vi "input.vi"(8 "error in":errorcluster, 10 "data table in":T1, 11 "TEC runtime in":refnum<class "TEC runtime.lvclass">) -> (0 "error out":errorcluster, 2 "data table out":T1, 3 "TEC runtime out":refnum<class "TEC runtime.lvclass">)   [LabVIEW 2013, in "TEC runtime.lvclass"]
doc: "Provides an interface for reading data from a module at runtime. While this interface performs no operations, a child should provide an override which may read from any open sessions, references, or interfaces."
uses:
  TEC runtime.lvclass
  <vilib>/NI/Tag Bus/table/data table.ctl
  TEC runtime.lvclass/TEC runtime.ctl
  <vilib>/NI/Tag Bus/table/data table.lvlib
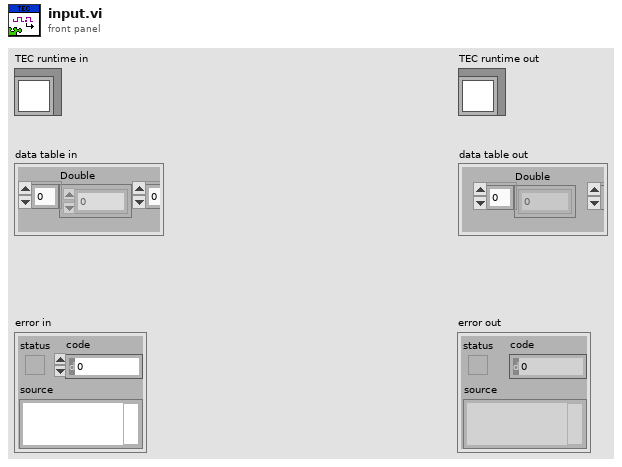
[diagram p1: front panel]
types:
  T1 = typedef "tag bus.lvlib/data table.lvlib/data table.ctl" = cluster{"Double":dbl[], "Single":sgl[], "I64":i64[], "I32":i32[], "I16":i16[], "I8":i8[], "U64":u64[], "U32":u32[], "U16":u16[], "U8":u8[], "Boolean":bool[], "String":string[], "Array of Double":cluster{"DBL Array":dbl[]}[], "Array of Single":cluster{"SGL Array":sgl[]}[], "Array of I64":cluster{"I64 Array":i64[]}[], "Array of I32":cluster{"I32 Array":i32[]}[], "Array of I16":cluster{"I16 Array":i16[]}[], "Array of I8":cluster{"I8 Array":i8[]}[], "Array of U64":cluster{"U64 Array":u64[]}[], "Array of U32":cluster{"U32 Array":u32[]}[], "Array of U16":cluster{"U16 Array":u16[]}[], "Array of U8":cluster{"U8 Array":u8[]}[], "Array of Boolean":cluster{"Boolean Array":bool[]}[], "Array of String":cluster{"String Array":string[]}[]}
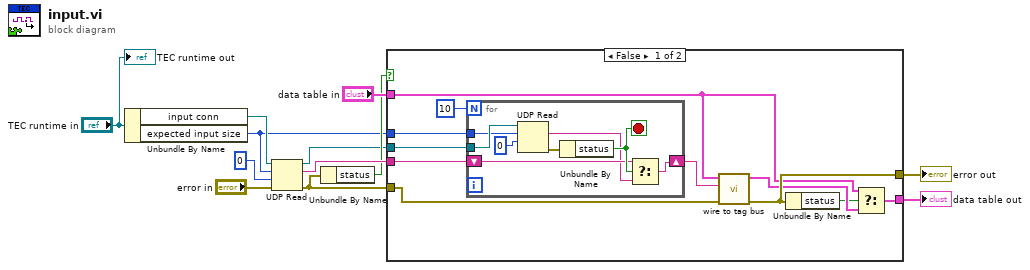
[diagram p0: block diagram]
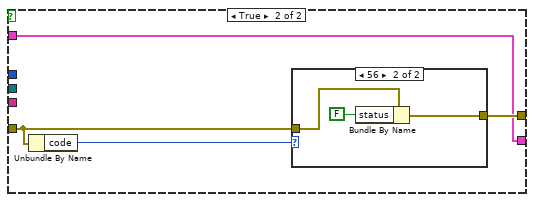
[diagram p2: hidden frame]
diagram:
  n1 = Unbundle By Name("TEC runtime in") -> ("input conn"=w11:refnum<k16>, "expected input size"=w1:i32)
  n2 = UDP Read(connection ID=w11, max size (548)=w1, timeout ms (25000)=0, 8:"error in") -> (data out=w5:string, error out=w3:errorcluster, 3:w2:refnum<k16>)  [unwired: 2 out]
  n3 = Unbundle By Name(w3) -> ("status"=w4:bool)
  n4 = case shown="False" w4 {
    tunnel: "data table in" -> [w20 w32]
    tunnel: [w23 w33] -> w7
    tunnel: [w21 w32] -> w6
    tunnel: w5 -> [w18 _]
    tunnel: w3 -> [w13 w34]
    tunnel: w2 -> [w15 _]
    tunnel: w1 -> [w14 _]
    frame False {
      n5 = for {
        N: 10 -> [_]
        shift-right: [w25] -> w17
        shift-left: w18 -> [w26]
        tunnel: w15 -> [w31]
        tunnel: w14 -> [w30]
        stop <- w27 stop-if-true
        n6 = UDP Read(connection ID=w31, max size (548)=w30, timeout ms (25000)=0) -> (data out=w24:string, error out=w28:errorcluster)  [unwired: 1 in, 3 out]
        n7 = Unbundle By Name(w28) -> ("status"=w27:bool)
        n8 = Select(t=w26, s=w27, f=w24) -> (s? t:f=w25:string)
      }
      n9 = call "wire to tag bus.vi"("error in"=w13, "wire data"=w17, "data table in"=w20) -> ("error out"=w23:errorcluster, "data table out"=w22:T1)  [unwired: 7 in]
      n10 = Unbundle By Name(w23) -> ("status"=w16:bool)
      n11 = Select(t=w20, s=w16, f=w22) -> (s? t:f=w21:T1)
    }
    frame True {
      n12 = Unbundle By Name(w34) -> ("code"=w35:i32)
      n13 = case shown="56" w35 {
        tunnel: w34 -> [w36 w39]
        tunnel: [w36 w37] -> w33
        frame Default {
        }
        frame 56 {
          n14 = Bundle By Name(cluster=w39, "status"=FALSE) -> (w37:errorcluster)
        }
      }
    }
  }
  "error out" <- w7
  "data table out" <- w6
  "TEC runtime out" <- "TEC runtime in"
